vi "CTR_ReadStatus.vi"(7 "DeviceIndex":u32, 8 "error in (no error)":errorcluster) -> (0 "error out":errorcluster)   [LabVIEW 2012]
doc: "unsigned long CTR_8254ReadStatus(\nunsigned long DeviceIndex - number from 0-31 indicating on which device you wish to read an\n8254 counter\nunsigned long BlockIndex - number indicating which 8254 you wish to read\nunsigned long CounterIndex - number from 0-2 indicating which counter on the specified 8254\nyou wish to read\nunsigned short *pReadValue - a pointer to a WORD in which will be stored the value latched\nand read from the specified counter\nunsigned char *pStatus - a pointer to a BYTE in which will be stored the status latched and read\nfrom the specified counter\n)"
uses:
  Windows/System32/AIOUSB.dll
panel:
  out "pStatus":u32
  out "pReadValue":u16
  in  "CounterIndex":u32
  in  "BlockIndex":u32
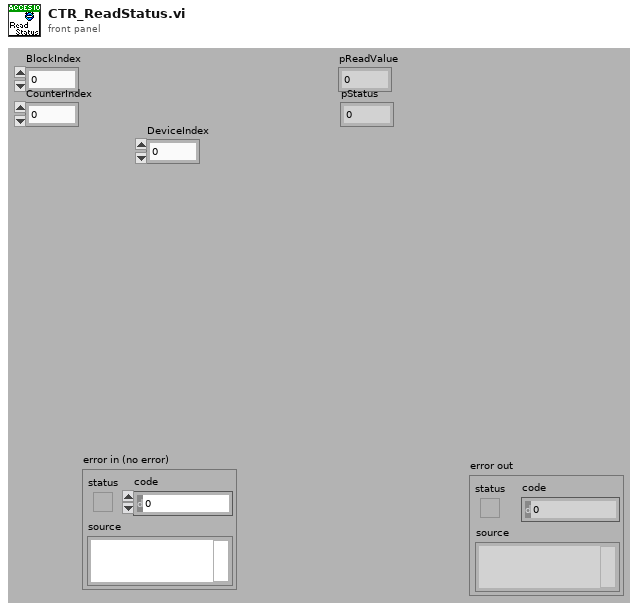
[diagram p1: front panel]
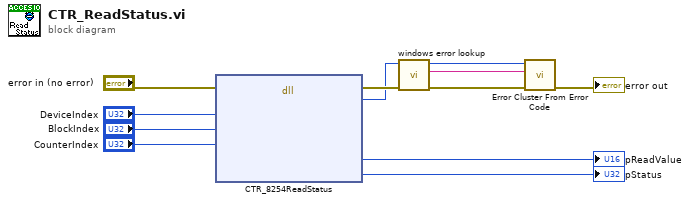
[diagram p0: block diagram]
diagram:
  n1 = dll-call lib="C:/Windows/System32/AIOUSB.dll" fn="CTR_8254ReadStatus"(error in="error in (no error)", "DeviceIndex"="DeviceIndex", "BlockIndex"="BlockIndex", "CounterIndex"="CounterIndex") -> (error out=w8:errorcluster, "return type"=w7:u32, "pReadValue"=→"pReadValue":u16, "pStatus"=→"pStatus":u32)  [unwired: 7 in, 1 out]
  n2 = call "windows error lookup.vi"("error in (no error)"=w8, "Error Code"=w7) -> ("error out"=w10:errorcluster, "error message (\"\")"=w11:string)  [unwired: 8 in]
  n3 = call <vilib>:"Error Cluster From Error Code.vi"("error in (no error)"=w10, "error message (\"\")"=w11, "error code (0)"=w7) -> ("error out"=→"error out":errorcluster)  [unwired: 6 in]
